vi "Add Device.vi"(10 "New Device":T1, 11 "ItemNames":string[][](array[string])) -> (3 "Updated ItemNames":string[][](array[string]))   [LabVIEW 2013, in "ACNET Devices Editor.lvlib"]
uses:
  ACNET Devices Editor.lvlib
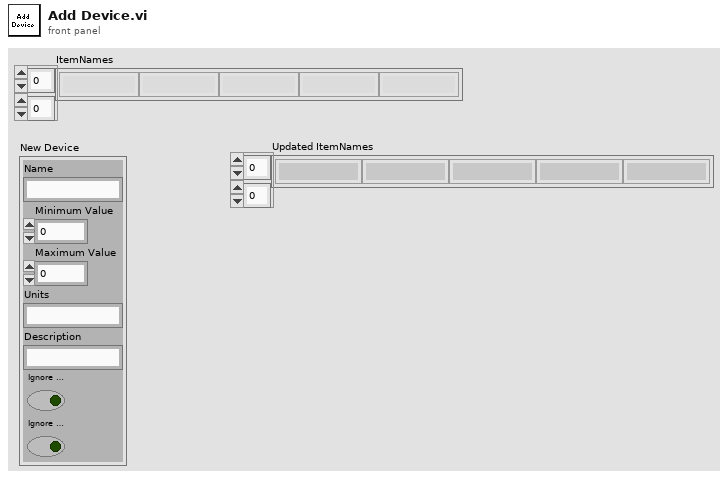
[diagram p1: front panel]
types:
  T1 = cluster{"Name":string, "Minimum Value":dbl, "Maximum Value":dbl, "Units":string, "Description":string, "Ignore Min Value":bool, "Ignore Max Value":bool}
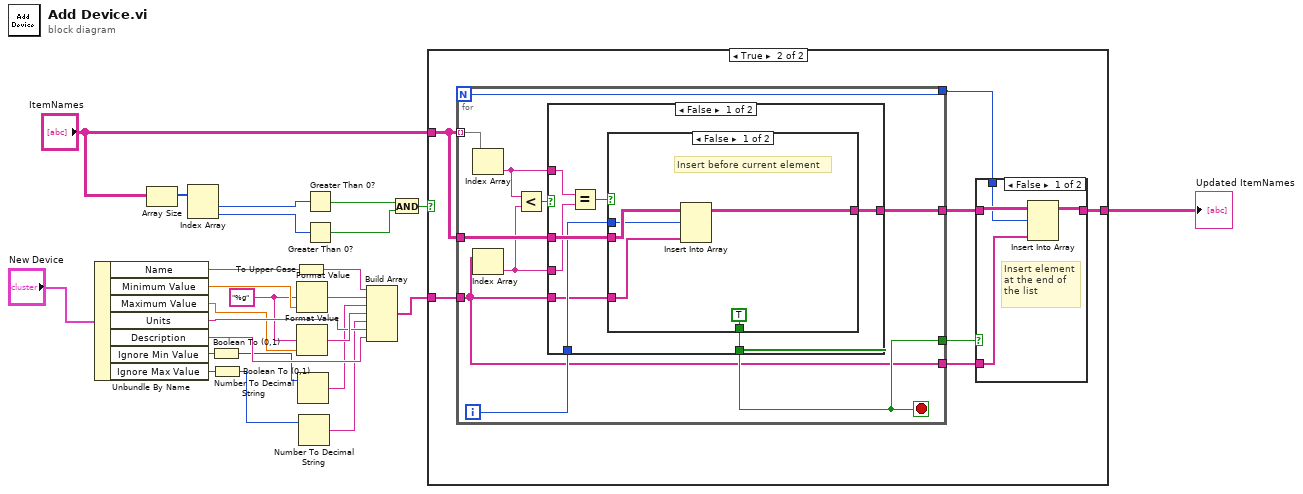
[diagram p0: block diagram]
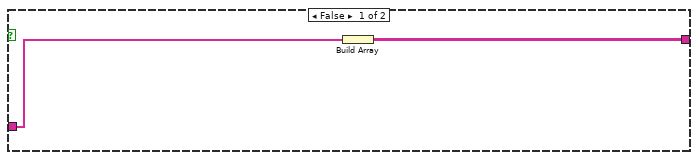
[diagram p2: hidden frame]
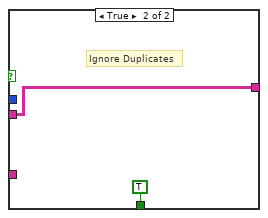
[diagram p4: hidden frame]
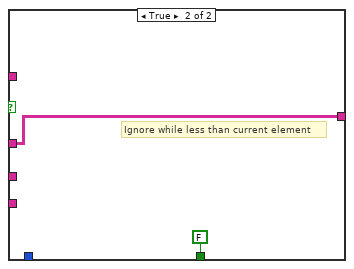
[diagram p5: hidden frame]
diagram:
  w1 = "%g" ("format string")
  n1 = Unbundle By Name("New Device") -> ("Name"=w14:string, "Minimum Value"=w3:dbl, "Maximum Value"=w2:dbl, "Units"=w11:string, "Description"=w10:string, "Ignore Min Value"=w9:bool, "Ignore Max Value"=w7:bool)
  n2 = Array Size(array="ItemNames") -> (size(s)=w22:i32[])
  n3 = Index Array(array=w22) -> (element #1=w20:i32, element #2=w19:i32)  [unwired: 2 in]
  n4 = Boolean To (0,1)(Boolean=w9) -> (0, 1=w8:i16)
  n5 = Boolean To (0,1)(Boolean=w7) -> (0, 1=w6:i16)
  n6 = To Upper Case(1:w14) -> (0:w13:string)
  n7 = Format Value(format string=w1, value (0)=w3) -> (output string=w15:string)  [unwired: 1 in]
  n8 = Format Value(format string=w1, value (0)=w2) -> (output string=w25:string)  [unwired: 1 in]
  n9 = Number To Decimal String(number=w8) -> (decimal integer string=w5:string)  [unwired: 1 in]
  n10 = Number To Decimal String(number=w6) -> (decimal integer string=w4:string)  [unwired: 1 in]
  n11 = Greater Than 0?(x=w20) -> (x > 0?=w17:bool)
  n12 = Greater Than 0?(x=w19) -> (x > 0?=w16:bool)
  n13 = Build Array(w13, w15, w5, w25, w4, w11, w10) -> (w24:string[])
  n14 = And(x=w17, y=w16) -> (x .and. y?=w18:bool)
  n15 = case shown="True" w18 {
    tunnel: "ItemNames" -> [_ w34]
    tunnel: w24 -> [w27 w31]
    tunnel: [w26 w29] -> w23
    frame False {
      n16 = Build Array(w27) -> (w26:string[][])
    }
    frame True {
      n17 = for {
        N -> [w40]
        tunnel: w34 -> [w48] mode=indexing
        tunnel: w34 -> [w46]
        tunnel: [w44] -> w32
        tunnel: [w43] -> w33
        tunnel: w31 -> [w41]
        tunnel: [w41] -> w30
        tunnel: [w40] -> w28
        i -> [w45]
        stop <- w43 stop-if-true
        n18 = Index Array(array=w48) -> (element=w47:string)  [unwired: 1 in]
        n19 = Index Array(array=w41) -> (element=w42:string)  [unwired: 1 in]
        n20 = Less?(x=w47, y=w42) -> (x < y?=w49:bool)
        n21 = case shown="False" w49 {
          tunnel: w47 -> [w57 _]
          tunnel: w42 -> [w51 _]
          tunnel: [w55 FALSE] -> w43
          tunnel: w46 -> [w54 w65]
          tunnel: w45 -> [w53 _]
          tunnel: [w52 w65] -> w44
          tunnel: w41 -> [w50 _]
          frame False {
            n22 = Equal?(x=w57, y=w51) -> (x = y?=w56:bool)
            n23 = case shown="False" w56 {
              tunnel: [TRUE TRUE] -> w55
              tunnel: w54 -> [w61 w63]
              tunnel: w53 -> [w60 _]
              tunnel: [w59 w63] -> w52
              tunnel: w50 -> [w58 _]
              frame False {
                # "Insert before current element"
                n24 = Insert Into Array(array=w61, index (row)=w60, new element=w58) -> (w59:string[][])  [unwired: 1 in]
              }
              frame True {
                # "Ignore Duplicates"
              }
            }
          }
          frame True {
            # "Ignore while less than current element"
          }
        }
      }
      n25 = case shown="False" w33 {
        tunnel: w32 -> [w37 w39]
        tunnel: [w36 w39] -> w29
        tunnel: w30 -> [w38 _]
        tunnel: w28 -> [w35 _]
        frame False {
          # "Insert element\nat the end of\nthe list"
          n26 = Insert Into Array(array=w37, index (row)=w35, new element=w38) -> (w36:string[][])  [unwired: 1 in]
        }
        frame True {
          # "Element was\nadded in loop"
        }
      }
    }
  }
  "Updated ItemNames" <- w23
